vi "save_config.vi"(8 "error in (no error)":errorcluster, 10 "Config Settings":T1, 11 "Path":path) -> (0 "error out":errorcluster)   [LabVIEW 2024]
uses:
  controls/Config_Settings.ctl
  <vilib>/Utility/config.llb/Write Key (Double).vi
  <vilib>/Utility/config.llb/Write Key (U32).vi
  <vilib>/Utility/config.llb/NI_LVConfig.lvlib
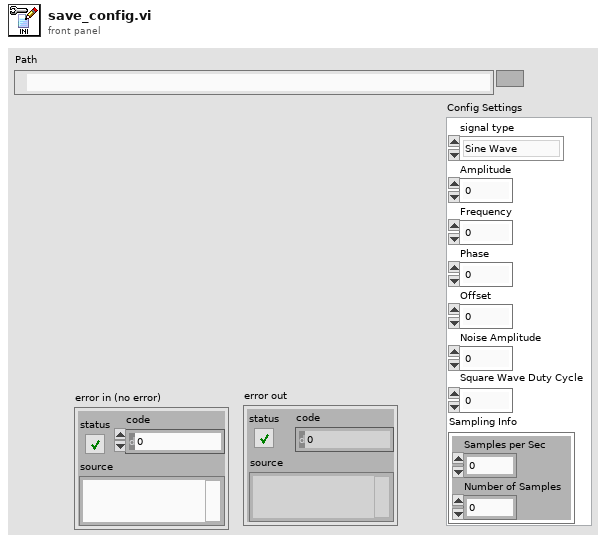
[diagram p1: front panel]
types:
  T1 = typedef "Config_Settings.ctl" = cluster{"signal type":enum16{"Sine Wave", "Triangle Wave", "Square Wave", "Sawtooth Wave"}, "Amplitude":dbl, "Frequency":dbl, "Phase":dbl, "Offset":dbl, "Noise Amplitude":dbl, "Square Wave Duty Cycle":dbl, "Sampling Info":cluster{"Samples per Sec":dbl, "Number of Samples":dbl}}
  T2 = enum16{"Sine Wave", "Triangle Wave", "Square Wave", "Sawtooth Wave"}
  T3 = typedef "NI_LVConfig.lvlib/Config Data RefNum.ctl" = refnum<k1>
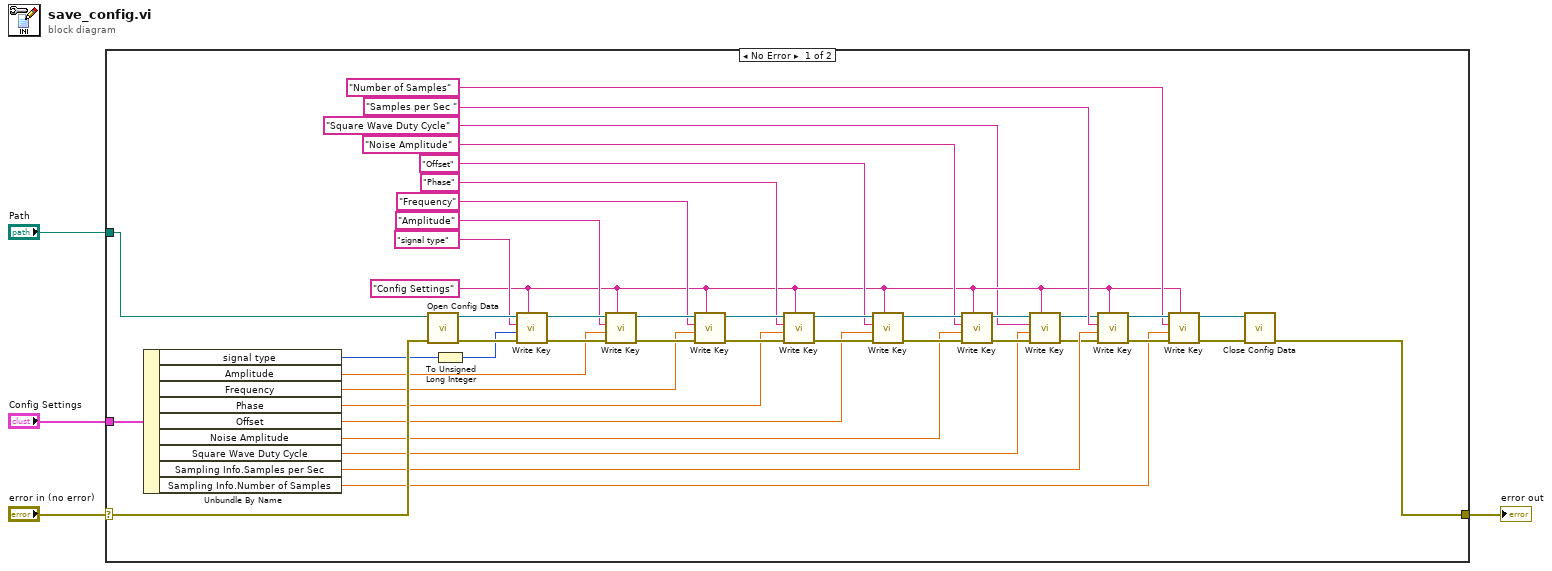
[diagram p0: block diagram]
diagram:
  n1 = case shown="No Error" "error in (no error)" {
    selector: "error in (no error)" -> [w40 w49]
    tunnel: [w41 w49] -> w3
    tunnel: "Path" -> [w33 _]
    tunnel: "Config Settings" -> [w48 _]
    frame No Error {
      w7 = "Config Settings" ("section")
      n2 = Unbundle By Name(w48) -> ("signal type"=w39:T2, "Amplitude"=w38:dbl, "Frequency"=w37:dbl, "Phase"=w36:dbl, "Offset"=w35:dbl, "Noise Amplitude"=w34:dbl, "Square Wave Duty Cycle"=w5:dbl, "Sampling Info.Samples per Sec"=w13:dbl, "Sampling Info.Number of Samples"=w12:dbl)
      n3 = call <vilib>:"Open Config Data.vi"("error in (no error)"=w40, "configuration file path"=w33) -> ("error out"=w47:errorcluster, "refnum"=w32:T3)  [unwired: 7 in, 1 out]
      n4 = To Unsigned Long Integer(number=w39) -> (unsigned 32bit integer=w26:u32)
      n5 = call-poly <vilib>:"Write Key.vi"("section"=w7, "error in (no error)"=w47, "value"=w26, "key"="signal type", "refnum"=w32) -> ("error out"=w46:errorcluster, "refnum out"=w31:T3)  [unwired: 4 in, 1 out]
      n6 = call-poly <vilib>:"Write Key.vi"("section"=w7, "error in (no error)"=w46, "value"=w38, "key"="Amplitude", "refnum"=w31) -> ("error out"=w45:errorcluster, "refnum out"=w30:T3)  [unwired: 4 in, 1 out]
      n7 = call-poly <vilib>:"Write Key.vi"("section"=w7, "error in (no error)"=w45, "value"=w37, "key"="Frequency", "refnum"=w30) -> ("error out"=w44:errorcluster, "refnum out"=w29:T3)  [unwired: 4 in, 1 out]
      n8 = call-poly <vilib>:"Write Key.vi"("section"=w7, "error in (no error)"=w44, "value"=w36, "key"="Phase", "refnum"=w29) -> ("error out"=w43:errorcluster, "refnum out"=w28:T3)  [unwired: 4 in, 1 out]
      n9 = call-poly <vilib>:"Write Key.vi"("section"=w7, "error in (no error)"=w43, "value"=w35, "key"="Offset", "refnum"=w28) -> ("error out"=w42:errorcluster, "refnum out"=w27:T3)  [unwired: 4 in, 1 out]
      n10 = call-poly <vilib>:"Write Key.vi"("section"=w7, "error in (no error)"=w42, "value"=w34, "key"="Noise Amplitude", "refnum"=w27) -> ("error out"=w11:errorcluster, "refnum out"=w9:T3)  [unwired: 4 in, 1 out]
      n11 = call-poly <vilib>:"Write Key.vi"("section"=w7, "error in (no error)"=w11, "value"=w5, "key"="Square Wave Duty Cycle", "refnum"=w9) -> ("error out"=w10:errorcluster, "refnum out"=w8:T3)  [unwired: 4 in, 1 out]
      n12 = call-poly <vilib>:"Write Key.vi"("section"=w7, "error in (no error)"=w10, "value"=w13, "key"="Samples per Sec ", "refnum"=w8) -> ("error out"=w17:errorcluster, "refnum out"=w19:T3)  [unwired: 4 in, 1 out]
      n13 = call-poly <vilib>:"Write Key.vi"("section"=w7, "error in (no error)"=w17, "value"=w12, "key"="Number of Samples", "refnum"=w19) -> ("error out"=w18:errorcluster, "refnum out"=w16:T3)  [unwired: 4 in, 1 out]
      n14 = call <vilib>:"Close Config Data.vi"("error in (no error)"=w18, "refnum"=w16) -> ("error out"=w41:errorcluster)  [unwired: 8 in, 1 out]
    }
    frame Error {
    }
  }
  "error out" <- w3
